vi "Heat1D_PreProcess BC.vi"(10 "Coefficients":cluster{"r":dbl, "s":dbl, "dt":dbl, "dx":dbl}, 11 "Boundary Condition":cluster{"type":T1, "Value":dbl[]}[](array[cluster]) {"type" items=["Dirichlet", "Neumann"]}) -> (1 "BC Type":i32, 2 "Right BC out":dbl[](array[numeric]), 3 "Left BC out":dbl[](array[numeric]))   [LabVIEW 2020, in "NI_PDE.lvlib"]
uses:
  <vilib>/gmath/NI_PDE.lvlib
  <vilib>/gmath/pde.llb/Common/PDE_BC Type.ctl
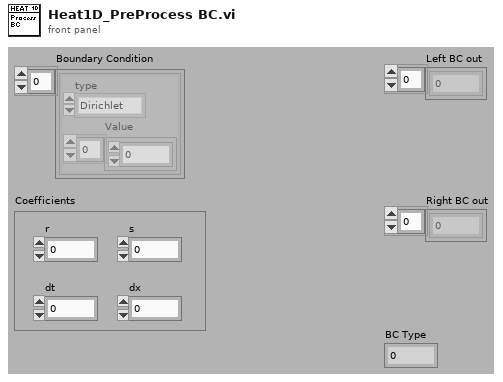
[diagram p1: front panel]
types:
  T1 = typedef "NI_PDE.lvlib/PDE_BC Type.ctl" = i32
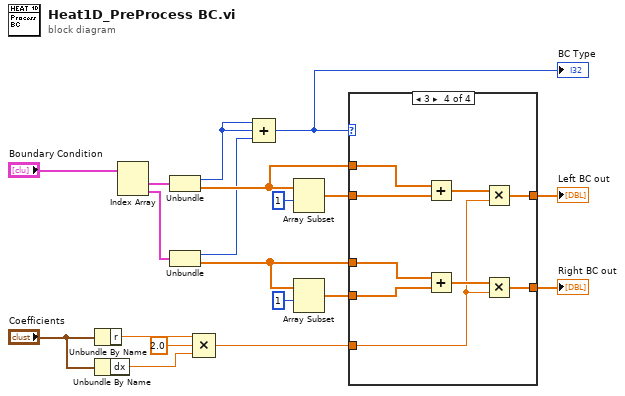
[diagram p0: block diagram]
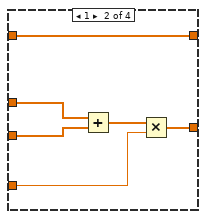
[diagram p3: hidden frame]
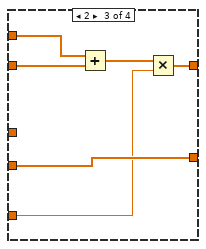
[diagram p4: hidden frame]
diagram:
  n1 = Unbundle By Name("Coefficients") -> ("r"=w6:dbl)
  n2 = Unbundle By Name("Coefficients") -> ("dx"=w3:dbl)
  n3 = Index Array(array="Boundary Condition") -> (element #1=w12:cluster{"type":T1, "Value":dbl[]}, element #2=w11:cluster{"type":T1, "Value":dbl[]})  [unwired: 2 in]
  n4 = Unbundle(w12) -> ("type"=w7:T1, "Value"=w10:dbl[])
  n5 = Unbundle(w11) -> ("type"=w8:T1, "Value"=w9:dbl[])
  n6 = Compound Arithmetic op=MULTIPLY(w6, 2.0 ("value"), w3) -> (w2:dbl)
  n7 = Compound Arithmetic op=ADD(w7, w7, w8) -> (w1:T1)
  "BC Type" <- w1
  n8 = Array Subset(array=w10, index=1) -> (w17:dbl[])  [unwired: 1 in]
  n9 = Array Subset(array=w9, index=1) -> (w16:dbl[])  [unwired: 1 in]
  n10 = case shown="3" w1 {
    tunnel: [w21 w25 w29 w34] -> w18
    tunnel: [w20 w22 w31 w38] -> w19
    tunnel: w17 -> [w21 w25 w32 w42]
    tunnel: w16 -> [w20 w26 w31 w40]
    tunnel: w10 -> [_ _ w33 w41]
    tunnel: w9 -> [_ w27 _ w39]
    tunnel: w2 -> [_ w23 w28 w35]
    frame 0, Default {
    }
    frame 1 {
      n11 = Add(x=w27, y=w26) -> (x+y=w24:dbl[])
      n12 = Multiply(x=w24, y=w23) -> (x*y=w22:dbl[])
    }
    frame 2 {
      n13 = Add(x=w33, y=w32) -> (x+y=w30:dbl[])
      n14 = Multiply(x=w30, y=w28) -> (x*y=w29:dbl[])
    }
    frame 3 {
      n15 = Add(x=w41, y=w42) -> (x+y=w36:dbl[])
      n16 = Add(x=w39, y=w40) -> (x+y=w37:dbl[])
      n17 = Multiply(x=w36, y=w35) -> (x*y=w34:dbl[])
      n18 = Multiply(x=w37, y=w35) -> (x*y=w38:dbl[])
    }
  }
  "Right BC out" <- w19
  "Left BC out" <- w18
